vi "Create New Report.vi"(8 "error in (no error)":errorcluster, 11 "Formatter in":refnum<class "Formatter.lvclass">) -> (0 "error out":errorcluster, 3 "Formatter out":refnum<class "Formatter.lvclass">)   [LabVIEW 2015, in "Formatter.lvclass"]
uses:
  Formatter.lvclass
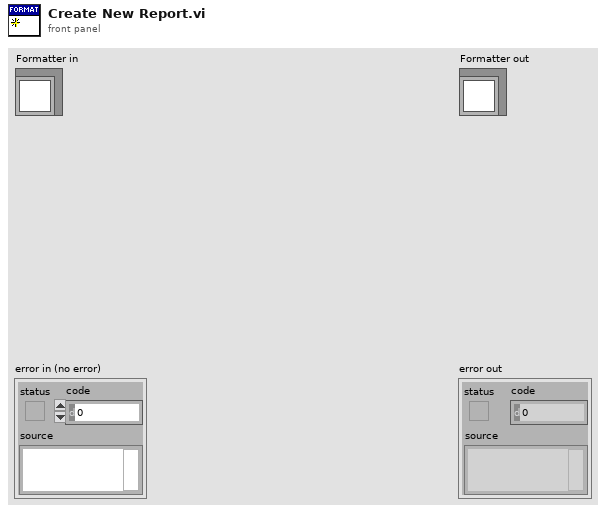
[diagram p1: front panel]
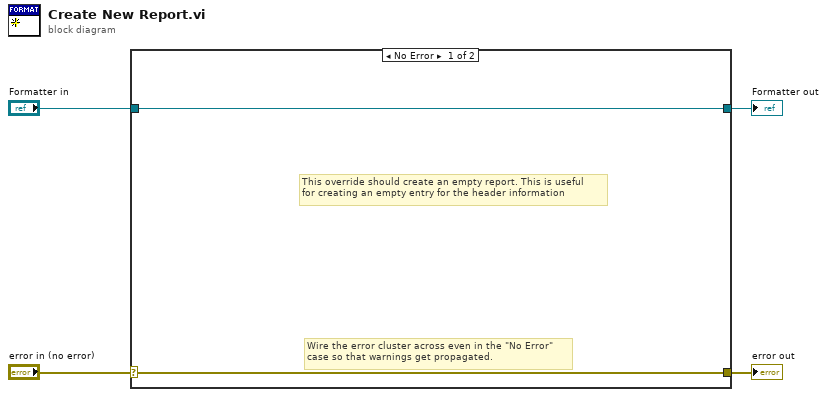
[diagram p0: block diagram]
diagram:
  n1 = case shown="No Error" "error in (no error)" {
    selector: "error in (no error)" -> [w5 w8]
    tunnel: [w5 w8] -> w3
    tunnel: [w6 w7] -> w1
    tunnel: "Formatter in" -> [w6 w7]
    frame No Error {
      # "This override should create an empty report. This is useful\nfor creating an empty entry for the header information"
      # "Wire the error cluster across even in the \"No Error\"\ncase so that warnings get propagated."
    }
    frame Error {
    }
  }
  "error out" <- w3
  "Formatter out" <- w1
